vi "ODE-DiseaseRHS.vi"(2 "data":variant, 3 "t":dbl, 4 "x1, x2,...":dbl[](array[numeric])) -> (0 "error out":errorcluster, 1 "f'(x)":dbl[](array[numeric]))   [LabVIEW 2023]
doc: "This VI contains the formula of the Communicable Disease ODE system model to be called by reference by the polymorphic ODE solver in VI mode. The Communicable Disease system can be described by the following equations:\n\nds/dt =-k1si\ndi/dt = -k2i + k1si\ndr/dt = k2i\n\nIn these equations, s(t), i(t), r(t) are the populations of those susceptible to, infected by, and recovered from the disease, respectively. The variable k1 is the infection rate, and k2 is the removal rate."
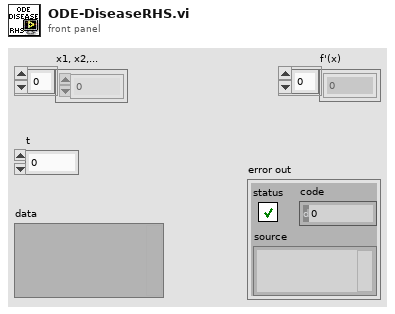
[diagram p1: front panel]
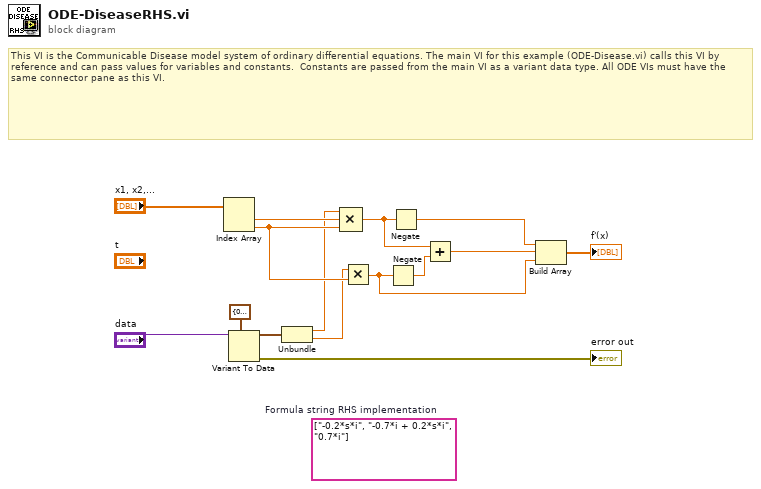
[diagram p0: block diagram]
diagram:
  (unwired) string[] ["-0.2*s*i", "-0.7*i + 0.2*s*i", "0.7*i"]  # Formula string RHS implementation
  # "This VI is the Communicable Disease model system of ordinary differential equations. The main VI for this example (ODE-Disease.vi) calls this VI by reference and can pass values for variables and constants.  Constants are passed from the main VI as a variant data type. All ODE VIs must have the same connector pane as this VI."
  n1 = Index Array(array="x1, x2,...") -> (element #1=w14:dbl, element #2=w10:dbl)  [unwired: 2 in]
  n2 = Variant To Data(type=cluster{"x":dbl, "x":dbl} {"x"=0.0, "x"=0.0} ("output cluster"), Variant="data") -> (data=w11:cluster{"x":dbl, "x":dbl}, error out=→"error out":errorcluster)  [unwired: 1 in]
  n3 = Unbundle(w11) -> ("x"=w9:dbl, "x"=w4:dbl)
  n4 = Compound Arithmetic op=MULTIPLY(w9, w14, w10) -> (w8:dbl)
  n5 = Multiply(x=w4, y=w10) -> (x*y=w3:dbl)
  n6 = Negate(x=w3) -> (-x=w5:dbl)
  n7 = Negate(x=w8) -> (-x=w6:dbl)
  n8 = Add(x=w8, y=w5) -> (x+y=w7:dbl)
  n9 = Build Array(w6, w7, w3) -> (→"f'(x)":dbl[])
